vi "new_unwarpping.vi"(11 "phase":dbl[](array[numeric])) -> (3 "unwrapped_phase":dbl[](array[numeric]))   [LabVIEW 2020]
uses:
  <vilib>/imath/engines/lvmath2/RunTimeEngine/BuiltInFunctions/size/NIMS_[I32,I32]=size(GRow).vi
  <instcachedir>/0/NIMS_[I32,I32]=size(GRow)_CFE2C4BDC5BC45CD88F2F6A295A2273D.lvgen/NIMS_[I32,I32]=size(GRow)_CFE2C4BDC5BC45CD88F2F6A295A2273D_000.vi
  <vilib>/imath/engines/lvmath2/RunTimeEngine/RangeToken/NIMS_Range_R2 - Integer.vi
  <instcachedir>/0/NIMS_Range_R2 - Integer_FEB7E399976F48268AE107D697ADF5D9.lvgen/NIMS_Range_R2 - Integer_FEB7E399976F48268AE107D697ADF5D9_000.vi
  <vilib>/imath/engines/lvmath2/RunTimeEngine/CommandStatement/MC_CommandStatement_break.vi
  <vilib>/imath/engines/lvmath2/RunTimeEngine/IndexRead/NIMS M(S,S).vi
  <instcachedir>/0/NIMS M(S,S)_AC51E74150A542F7991B9634C66F3096.lvgen/NIMS M(S,S)_AC51E74150A542F7991B9634C66F3096_000.vi
  <vilib>/imath/engines/lvmath2/RunTimeEngine/ErrorHandling/NIMS_Create Error From Enums.vi
  <vilib>/imath/engines/lvmath2/RunTimeEngine/IndexReplace/NIMS M(S,S)=S.vi
  <instcachedir>/0/NIMS M(S,S)=S_399908DFD004401BA66ACC94B4F53E50.lvgen/NIMS M(S,S)=S_399908DFD004401BA66ACC94B4F53E50_000.vi
  <vilib>/imath/engines/lvmath2/RunTimeEngine/NodeEndStatement/NIMS_NodeEndStatement_Get Vector.vi
  <instcachedir>/0/NIMS_NodeEndStatement_Get Vector_A95D2DB2A9BC46BA8CD6C6E4D7235685.lvgen/NIMS_NodeEndStatement_Get Vector_A95D2DB2A9BC46BA8CD6C6E4D7235685_001.vi
  <vilib>/imath/engines/lvmath2/RunTimeEngine/NodeEndStatement/NIMS_NodeEndStatement_Output.vi
  <instcachedir>/0/NIMS_NodeEndStatement_Output_53EC0D466D134D7ABD903AC30B43404B.lvgen/NIMS_NodeEndStatement_Output_53EC0D466D134D7ABD903AC30B43404B_005.vi
  <vilib>/imath/engines/lvmath2/RunTimeEngine/ErrorHandling/NIMS_Finalize Error.vi
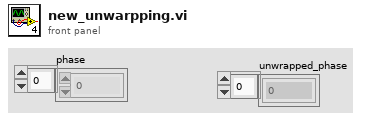
[diagram p1: front panel]
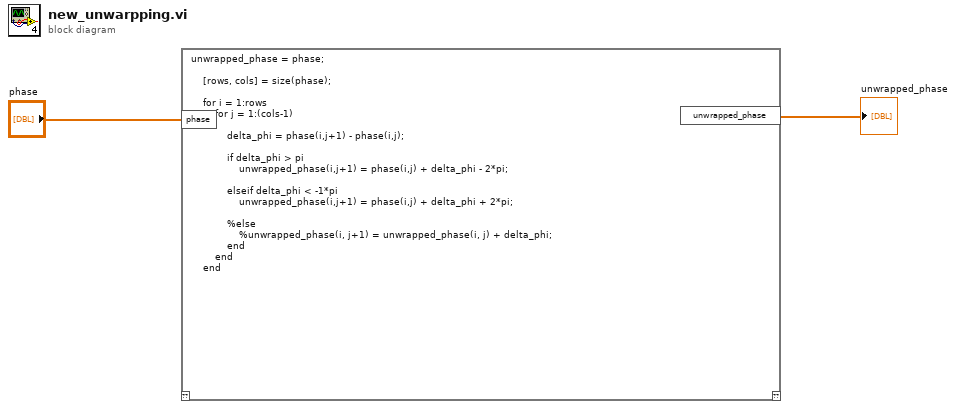
[diagram p0: block diagram]
diagram:
  n1 = mathscript code="unwrapped_phase = phase;\n    \n    [rows, cols] = size(phase);\n    \n    for i = 1:rows\n        for j = 1:(cols-1) \n\n            delta_phi = phase(i,j+1) - phase(i,j);\n            \n            if delta_phi > pi\n                unwrapped_phase(i,j+1) = phase(i,j) + delta_phi - 2*pi;\n\n            elseif delta_phi < -1*pi\n                unwrapped_phase(i,j+1) = phase(i,j) + delta_phi + 2*pi;\n\n            %else \n                %unwrapped_phase(i, j+1) = unwrapped_phase(i, j) + delta_phi;\n            end\n        end\n    end"("phase"="phase") -> ("unwrapped_phase"=→"unwrapped_phase":dbl[])  [unwired: 1 in, 1 out]
